vi "TimeToMatch.vi"() -> ()   [LabVIEW 2025]
panel:
  out "Time to Match":dbl[unit]
  out "# of iterations":i32
  out "Current Number":i32
  in  "Number to Match":i32
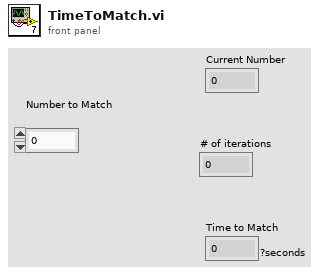
[diagram p1: front panel]
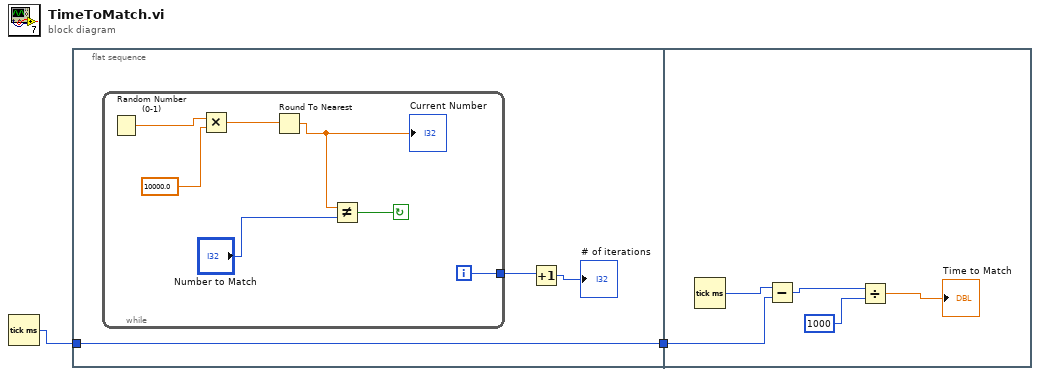
[diagram p0: block diagram]
diagram:
  n1 = Tick Count (ms)() -> (millisecond timer value=w2:u32)
  n2 = flat-sequence {
    tunnel: w2 -> [w3]
    tunnel: [w3] -> w1
    tunnel: w1 -> [w16]
    frame #0 {
      n3 = while {
        tunnel: [w8] -> w5
        i -> [w8]
        stop <- w6 continue-if-true
        n4 = Random Number (0-1)() -> (number: 0 to 1=w12:dbl)
        n5 = Multiply(x=w12, y=10000.0) -> (x*y=w10:dbl)
        n6 = Round To Nearest(number=w10) -> (nearest integer value=w9:dbl)
        "Current Number" <- w9
        n7 = Not Equal?(x=w9, y="Number to Match") -> (x != y?=w6:bool)
      }
      n8 = Increment(x=w5) -> (x+1=→"# of iterations":i32)
    }
    frame #1 {
      n9 = Tick Count (ms)() -> (millisecond timer value=w17:u32)
      n10 = Subtract(x=w17, y=w16) -> (x-y=w15:u32)
      n11 = Divide(x=w15, y=1000) -> (x/y=→"Time to Match":dbl)
    }
  }
